vi "DebugWebSerice.Async.vi"(10 "Parameters":variant, 11 "Process":refnum<class "Process.lvclass">) -> ()   [LabVIEW 2017, in "DebugWebSerice Engine.lvlib"]
uses:
  DebugWebSerice Engine.lvlib
  <vilib>/NI/NIVS Inline Async API/_VS Inline Async API/Process/Process.lvclass
  <vilib>/NI/NIVS Inline Async API/_VS Inline Async API/Process/Process.lvclass/Process.ctl
  <vilib>/NI/NIVS Inline Async API/_Data Access Engine/Access Type Classes/Read/Read.lvclass/Read.ctl
  <vilib>/NI/NIVS Inline Async API/_Data Access Engine/Access Type Classes/Write/Write.lvclass/Write.ctl
  <vilib>/NI/NIVS Inline Async API/_Data Access Engine/Data Access Engine/Methods/Read.Data.vi
  <vilib>/NI/NIVS Inline Async API/_Data Access Engine/Data Access Engine/Methods/Write.Data.vi
  <vilib>/NI/NIVS Inline Async API/_VS Inline Async API/Process/Data Member Access/Read Data Access.vi
  <vilib>/NI/NIVS Inline Async API/_VS Inline Async API/Error Handling Process/SubVIs/Error.ConvertArray.vi
  <vilib>/NI/NIVS Inline Async API/_Data Access Engine/Access Type Classes/Read/Read.ProcessData.vi
  <vilib>/NI/NIVS Inline Async API/_Data Access Engine/Access Type Classes/Write/Write.ProcessData.vi
  <vilib>/NI/NIVS Inline Async API/_Data Access Engine/Data Access Engine/Methods/Read.Lookup.vi
  <vilib>/NI/NIVS Inline Async API/_Data Access Engine/Data Access Engine/Methods/Write.Lookup.vi
  <vilib>/NI/NIVS Inline Async API/_Data Access Engine/Data Access Engine/Data Access Engine.lvclass
  source/vsws_api/vsws.lvlib
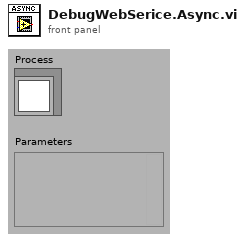
[diagram p1: front panel]
types:
  T1 = typedef "Data Access Engine.lvlib/Data Access Engine.lvclass/Write.DVR.ctl" = refnum<data-value>
  T2 = typedef "Data Access Engine.lvlib/Data Access Engine.lvclass/Read.DVR.ctl" = refnum<data-value>
  T3 = typedef "vsws.lvlib/cmdRef.ctl" = cluster{"queueRef":refnum<queue>, "reponseQueue":refnum<queue>}
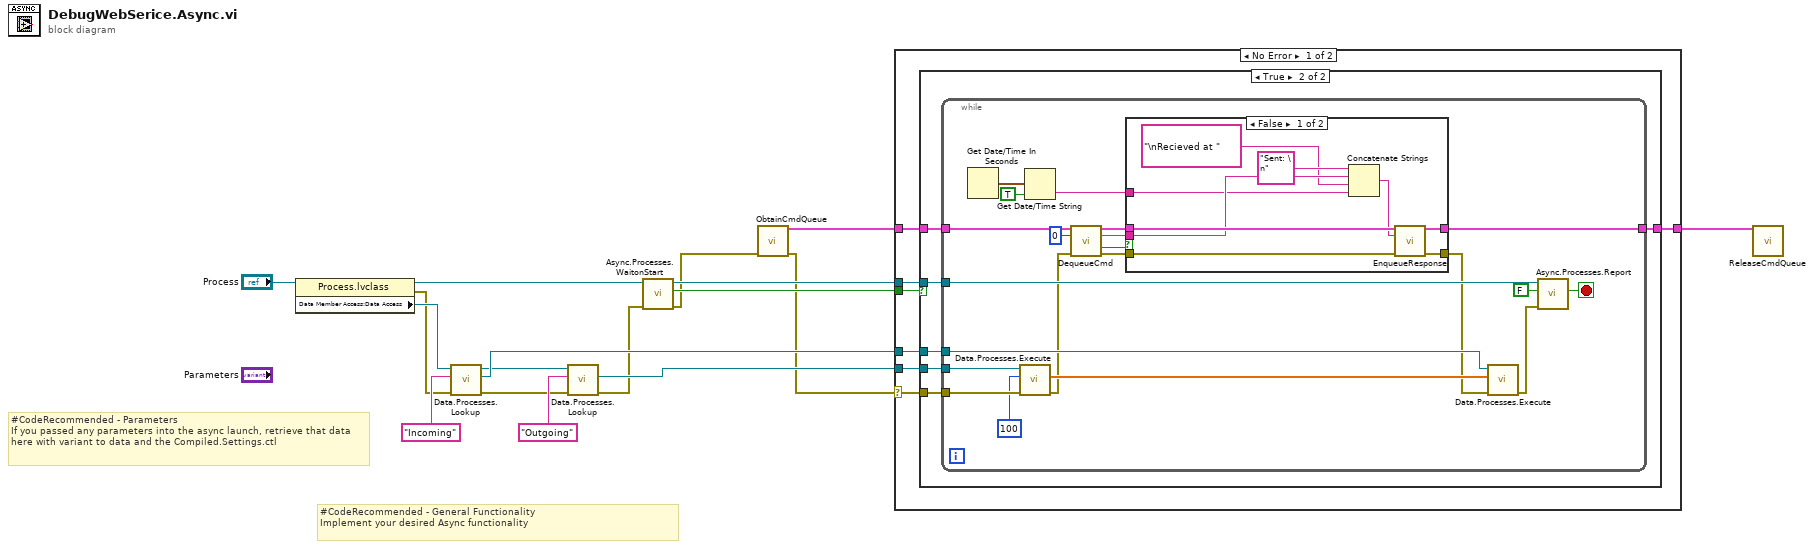
[diagram p0: block diagram]
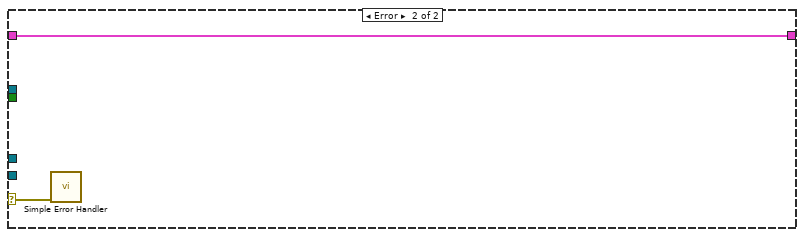
[diagram p4: hidden frame]
diagram:
  # "#CodeRecommended - General Functionality\nImplement your desired Async functionality"
  # "#CodeRecommended - Parameters\nIf you passed any parameters into the async launch, retrieve that data here with variant to data and the Compiled.Settings.ctl"
  n1 = property class="Process.lvclass"(reference="Process") -> (reference out=w7:refnum<class "Process.lvclass">, error out=w5:errorcluster, "Data Member Access:Data Access"=w6:refnum<class "Data Access Engine.lvclass">)  [unwired: 1 in]
  n2 = call-poly <vilib>:"Data.Processes.Lookup.vi"("error in (no error)"=w5, "Name"="Incoming", "Data Access API in"=w6) -> ("error out"=w12:errorcluster, "Ref"=w11:T1, "Data Access API out"=w10:refnum<class "Data Access Engine.lvclass">)  [unwired: 5 in, 1 out]
  n3 = call-poly <vilib>:"Data.Processes.Lookup.vi"("error in (no error)"=w12, "Name"="Outgoing", "Data Access API in"=w10) -> ("error out"=w9:errorcluster, "Ref"=w14:T2)  [unwired: 5 in, 2 out]
  n4 = call <vilib>:"Async.Processes.WaitonStart.vi"("error in (no error)"=w9, "Process"=w7) -> ("error out"=w4:errorcluster, "Execute"=w17:bool, "Process out"=w16:refnum<class "Process.lvclass">)  [unwired: 7 in]
  n5 = call "ObtainCmdQueue.vi"("error in (no error)"=w4) -> ("cmdRef"=w2:T3, "error out"=w3:errorcluster)  [unwired: 13 in]
  n6 = case shown="No Error" w3 {
    selector: w3 -> [w20 w65]
    tunnel: w17 -> [w24 _]
    tunnel: w16 -> [w23 _]
    tunnel: w11 -> [w22 _]
    tunnel: w14 -> [w21 _]
    tunnel: w2 -> [w19 w64]
    tunnel: [w18 w64] -> w1
    frame No Error {
      n7 = case shown="True" w24 {
        tunnel: w20 -> [_ w28]
        tunnel: w23 -> [_ w29]
        tunnel: w21 -> [_ w31]
        tunnel: w22 -> [_ w30]
        tunnel: w19 -> [w25 w27]
        tunnel: [w25 w26] -> w18
        frame False {
        }
        frame True {
          n8 = while {
            tunnel: w28 -> [w48]
            tunnel: w29 -> [w52]
            tunnel: w31 -> [w50]
            tunnel: w30 -> [w49]
            tunnel: w27 -> [w44]
            tunnel: [w36] -> w26
            stop <- w51 stop-if-true
            n9 = Get Date/Time In Seconds() -> (seconds since 1Jan1904=w40:timestamp)
            n10 = call-poly <vilib>:"Data.Processes.Execute.vi"("error in (no error)"=w48, "timeout ms"=100, "Ref"=w50) -> ("error out"=w43:errorcluster, "Values"=w46:dbl[])  [unwired: 6 in, 1 out]
            n11 = Get Date/Time String(seconds (now)=w40, want seconds? (F)=TRUE) -> (time string=w39:string)  [unwired: 1 in, 1 out]
            n12 = call "DequeueCmd.vi"("cmdRef in"=w44, "timeout in ms (-1)"=0, "error in (no error)"=w43) -> ("cmdRef out"=w42:T3, "postdata"=w41:string, "timed out?"=w34:bool, "error out"=w37:errorcluster)  [unwired: 9 in]
            n13 = case shown="False" w34 {
              tunnel: w42 -> [w61 w63]
              tunnel: w41 -> [w59 _]
              tunnel: w39 -> [w57 _]
              tunnel: w37 -> [w55 w62]
              tunnel: [w54 w63] -> w36
              tunnel: [w53 w62] -> w35
              frame False {
                n14 = Concatenate Strings("Sent: \n", w59, "\nRecieved at " ("string"), w57) -> (w56:string)
                n15 = call "EnqueueResponse.vi"("cmdRef in"=w61, "response"=w56, "error in (no error)"=w55) -> ("cmdRef out"=w54:T3, "error out"=w53:errorcluster)  [unwired: 11 in]
              }
              frame True {
              }
            }
            n16 = call-poly <vilib>:"Data.Processes.Execute.vi"("error in (no error)"=w35, "Values"=w46, "Ref"=w49) -> ("error out"=w45:errorcluster)  [unwired: 8 in]
            n17 = call <vilib>:"Async.Processes.Report.vi"("Error"=w45, "Stop Async on Error?"=FALSE, "Process in"=w52) -> ("Stop"=w51:bool)  [unwired: 7 in, 1 out]
          }
        }
      }
    }
    frame Error {
      n18 = call <vilib>:"Simple Error Handler.vi"("error in (no error)"=w65) -> ()  [unwired: 4 in, 5 out]
    }
  }
  n19 = call "ReleaseCmdQueue.vi"("cmdRef"=w1) -> ()  [unwired: 14 in, 1 out]
